vi "Ver 4.1.vi"() -> ()   [LabVIEW 2016]
doc: "This example VI shows how to use thermocouples to take a temperature measurement.\n\nNote:\nFor front panel measurements, make sure the Input switch is in the out position(F)\nFor plug-in card measurements, make sure the Input switch is in the in poisition(R)"
uses:
  Documents/keithley_27xx/Keithley 27XX/Public/Configure/Measurement Specific/Configure FRTD.vi
  Documents/keithley_27xx/Keithley 27XX/Public/Configure/Measurement Specific/Configure Thermocouple.vi
  Documents/keithley_27xx/Keithley 27XX/Public/Configure/Measurement Specific/Configure Thermistor.vi
  Documents/keithley_27xx/Keithley 27XX/Public/Data/Read Multiple Direct.vi
  <vilib>/Utility/file.llb/Write Delimited Spreadsheet (DBL).vi
  Documents/keithley_27xx/Keithley 27XX/Keithley 27XX.lvlib
panel:
  in  "Delay (s)":dbl
  in  "Notes":string
  in  "Number of Channels\nMeasured":dbl=3.0
  in  "Sensor Name 2":string
  in  "Sensor Name 1":string
  in  "Sensor Name 0":string
  out "XY Graph":cluster{dbl[], dbl[]}[](graph)
  out "Timestamp 2":dbl[](array[numeric])
  out "Timestamp 1":dbl[](array[numeric])
  out "Timestamp 0":dbl[](array[numeric])
  out "Case 2":dbl[](array[numeric])
  out "Case 1":dbl[](array[numeric])
  in  "Channel (2)":string="103"
  in  "Alpha2":dbl=0.0038
  in  "Beta2":dbl=0.1
  in  "Delta2 3":dbl=1.0
  in  "Sensor Type 2":string(combo)="Thermistor"
  in  "Channel (1)":string="102"
  in  "Alpha1":dbl=0.0038
  in  "Beta1":dbl=0.1
  in  "Delta1 2":dbl=1.0
  in  "Sensor Type 1":string(combo)="Thermistor"
  in  "Sensor Type 0":string(combo)="Thermistor"
  in  "Delta0":dbl=1.0
  in  "Beta0":dbl=0.1
  in  "Alpha0":dbl=0.0038
  in  "Serial Configuration":T1={"Baud Rate (9600)"=9600, "Flow Control (1: XON/XOFF)"=1, "Termination Char (0:CR)"=0} {"Termination Char (0:CR)" items=["CR", "LF", "CRLF (Do not use)", "LFCR (Do not use)"]; "Flow Control (1: XON/XOFF)" items=["None", "XON/XOFF", "RTS/CTS (2701 Only)", "XON/XOFF & RTS/CTS (2701 Only)"]; "Baud Rate (9600)" items=["300"=300, "600"=600, "1200"=1200, "2400"=2400, "4800"=4800, "9600"=9600, "19.2k"=19200, "38.4k (2701 Only)"=38400, "57.6k (2701 Only)"=57600, "115.2k (2701 Only)"=115200]}
  in  "VISA resource name":refnum<visa-resource-name>="TCPIP0::192.168.69.200::1394::SOCKET"
  in  "stop":bool
  out "Case 0":dbl[](array[numeric])
  in  "Channel (0)":string="101"
  in  "Temperature (0: Celsius)":u16(ring) items=["Celsius", "Fahrenheit", "Kelvin"]
  # "This is the delay in seconds \nbetween measuring. Note \nthat 0 is the fastest setting"
  # "Use this stop unless it is an emergency.\nUse the stop sign in the tool bar if \nthere is a danger from proceeding."
  # "*For front panel measurements, make sure the Input switch is in the out position(F)*\n  For plug-in card measurements, make sure the Input switch is in the in position(R)"
  # "© 2005 National Instruments Corporation.  ALL RIGHTS RESERVED."
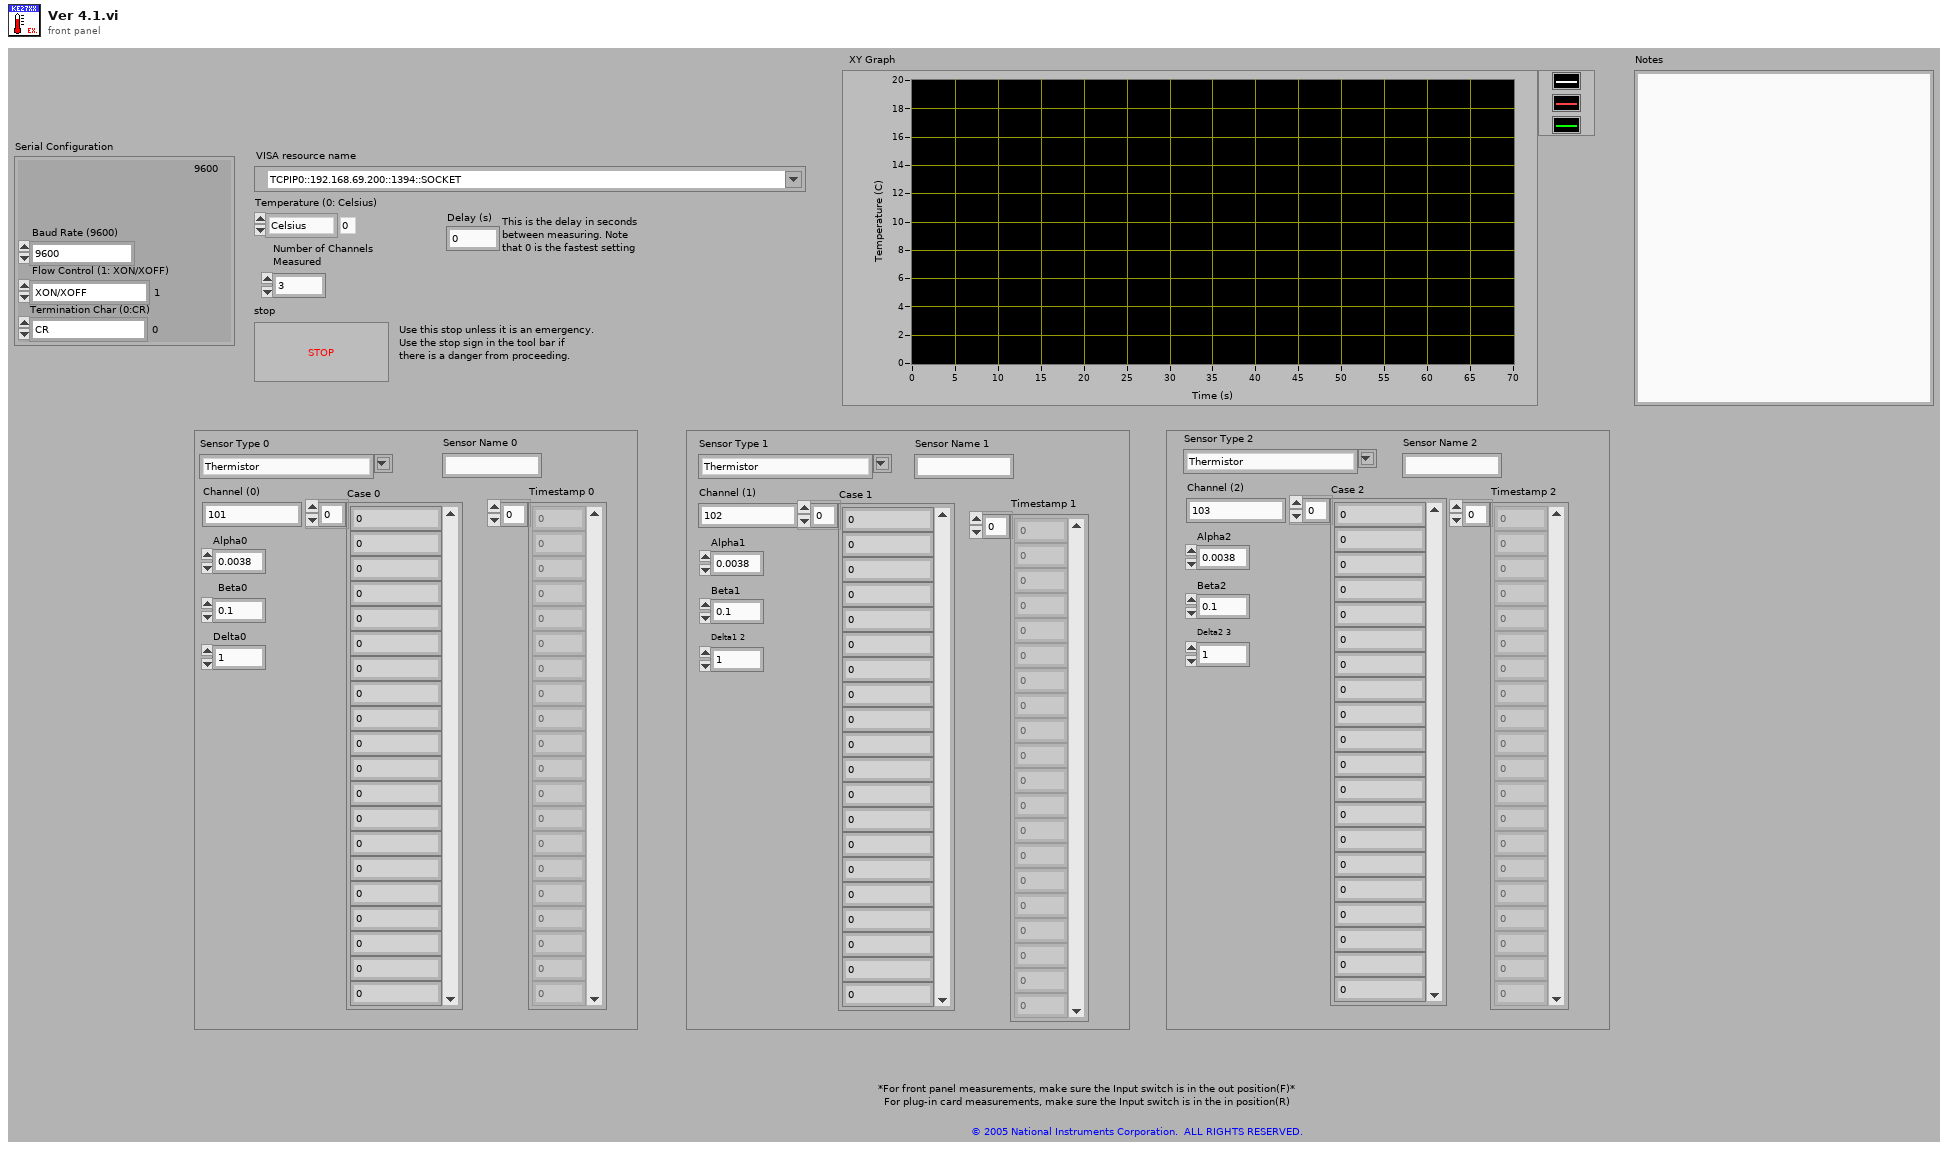
[diagram p1: front panel]
types:
  T1 = cluster{"Baud Rate (9600)":u32, "Flow Control (1: XON/XOFF)":u16, "Termination Char (0:CR)":u16}
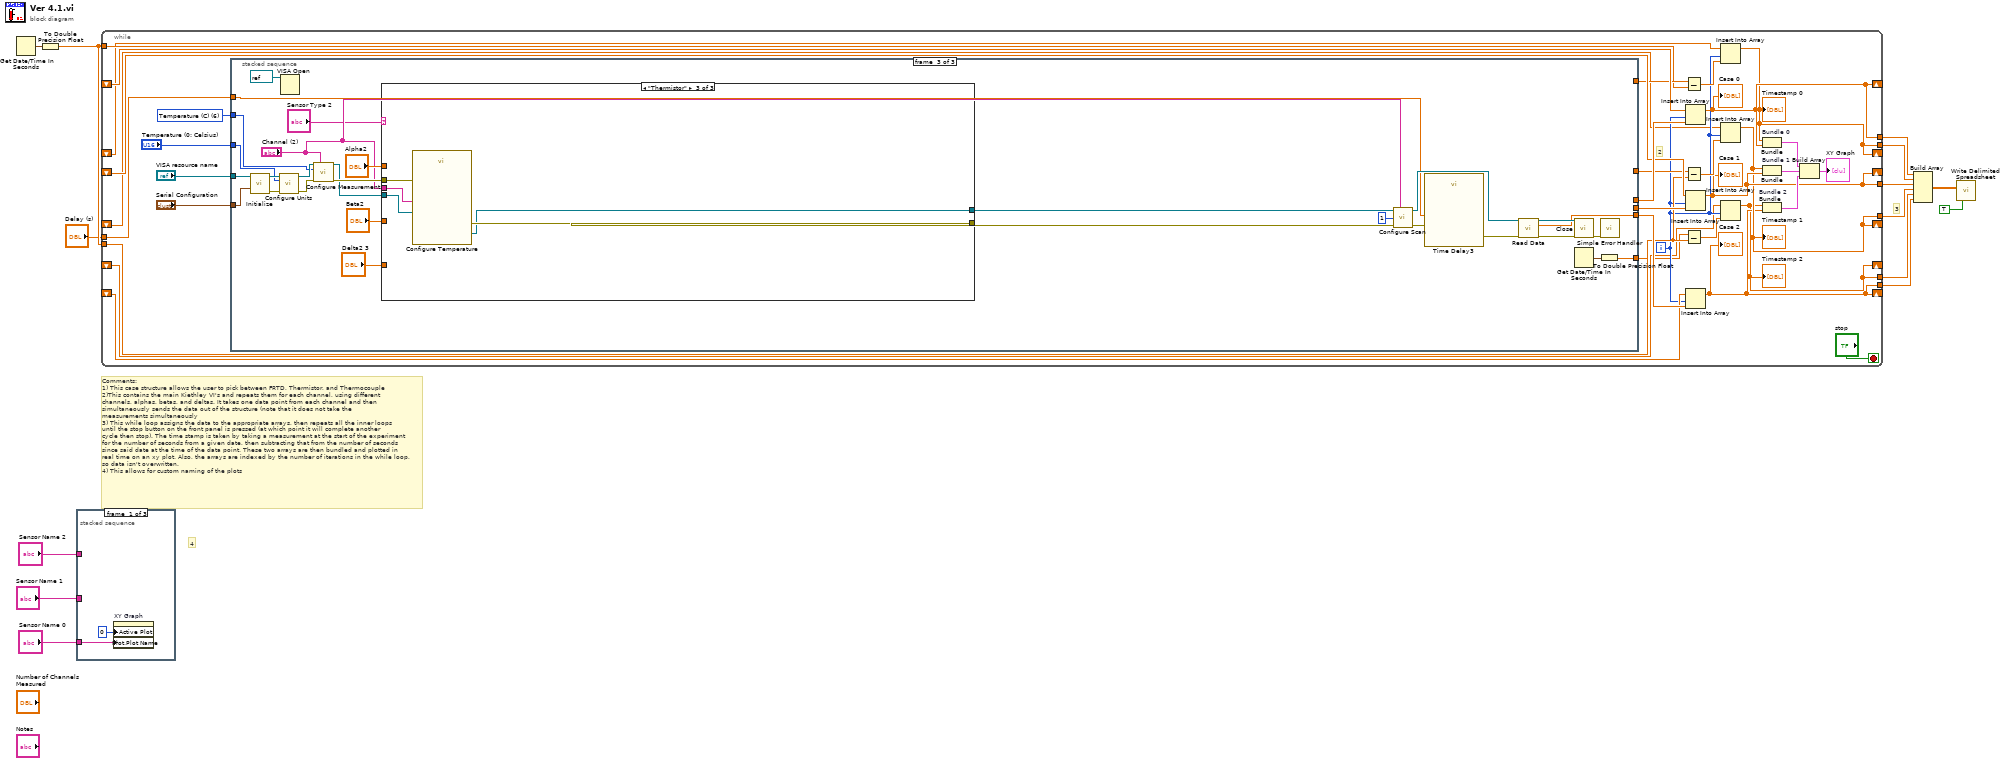
[diagram p0: block diagram]
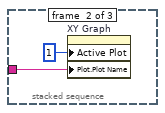
[diagram p2: hidden frame]
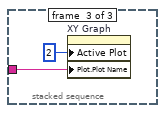
[diagram p3: hidden frame]
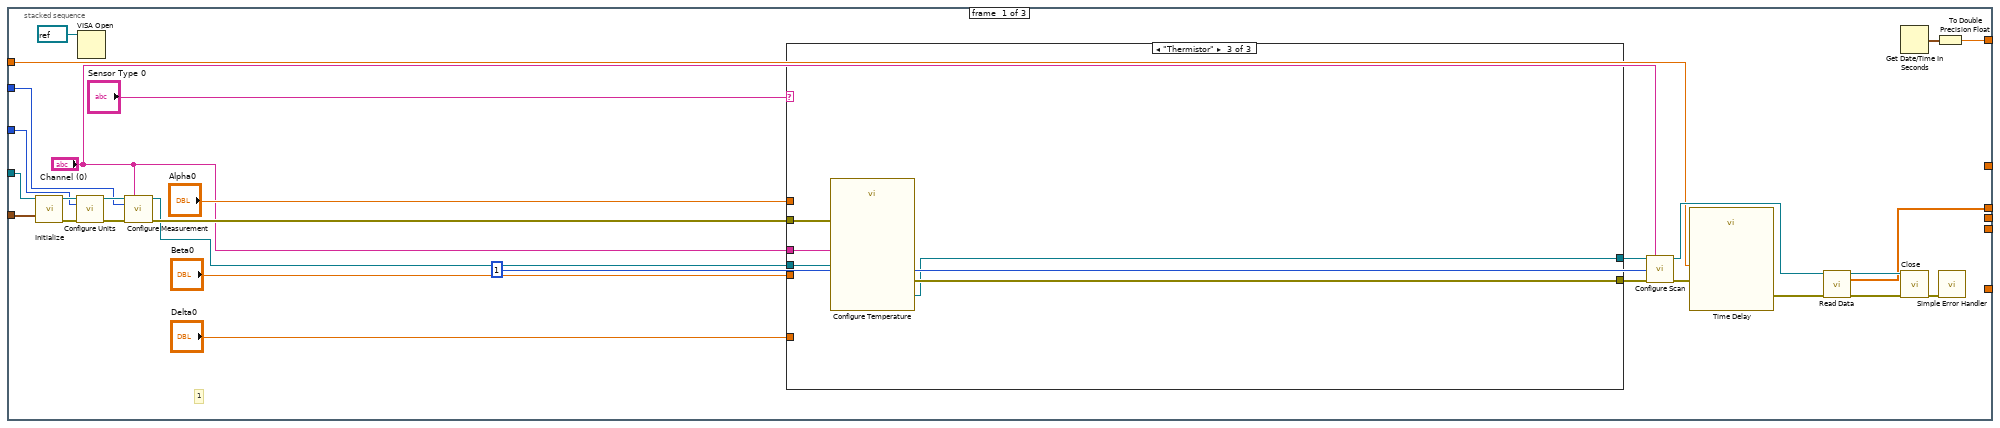
[diagram p4: hidden frame]
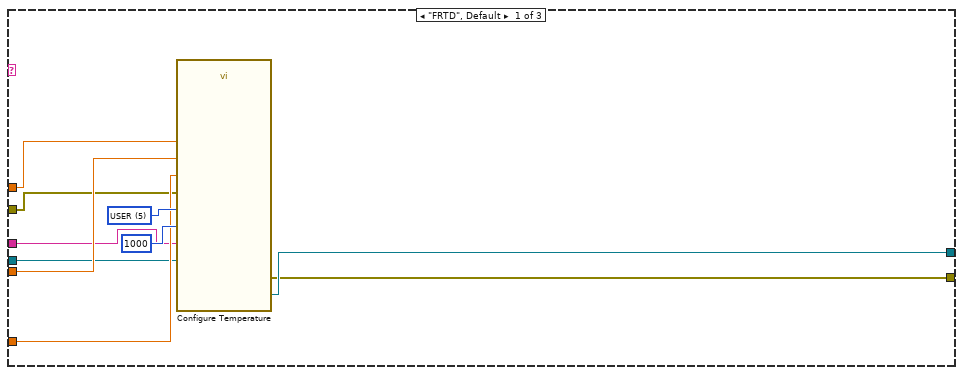
[diagram p5: hidden frame]
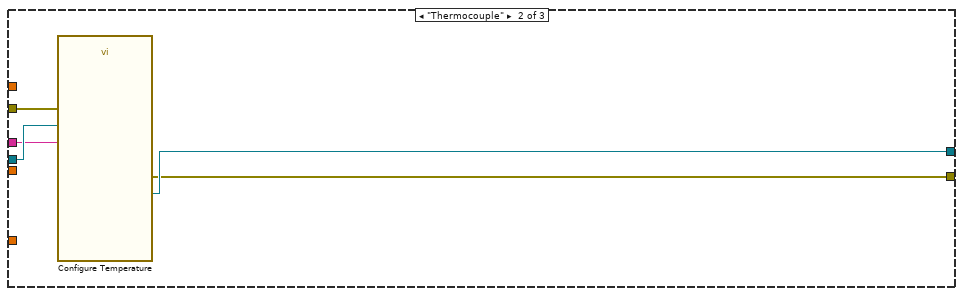
[diagram p6: hidden frame]
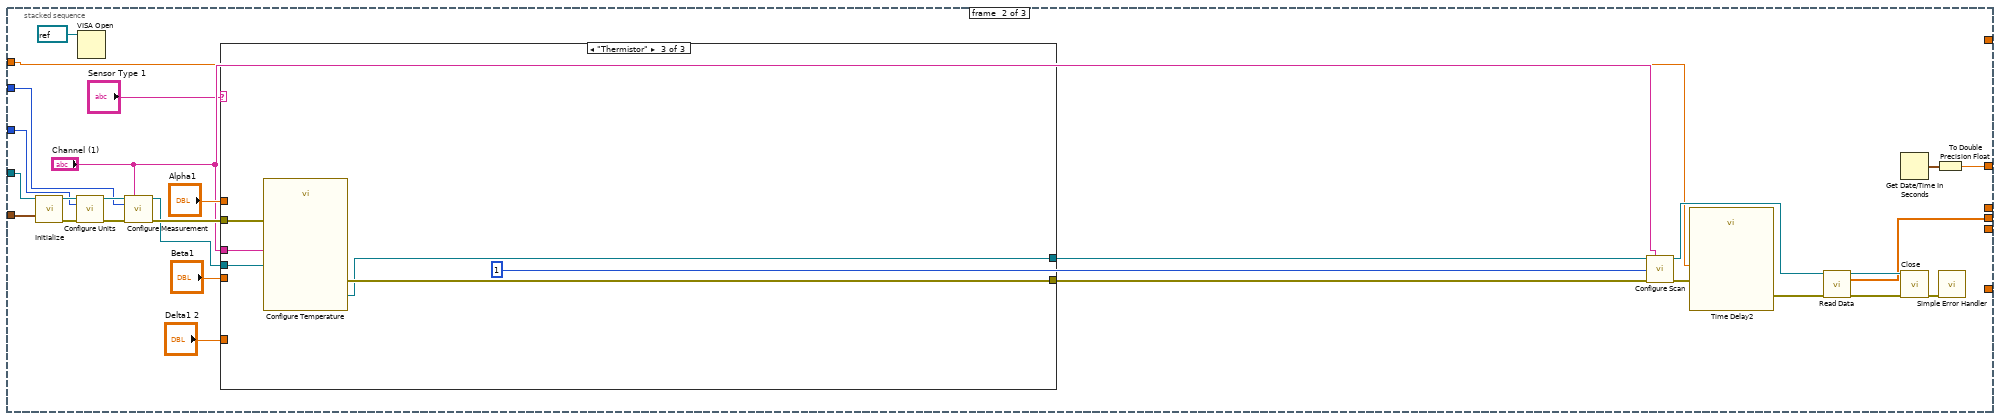
[diagram p7: hidden frame]
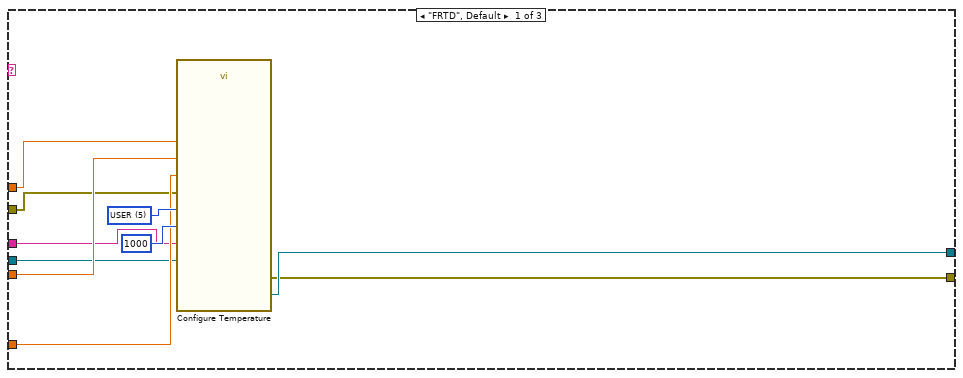
[diagram p8: hidden frame]
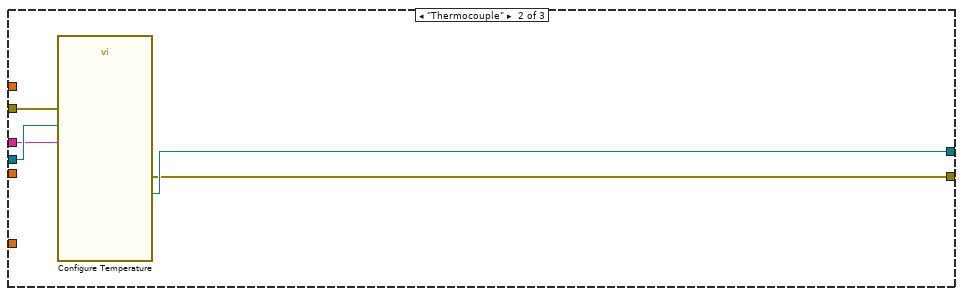
[diagram p9: hidden frame]
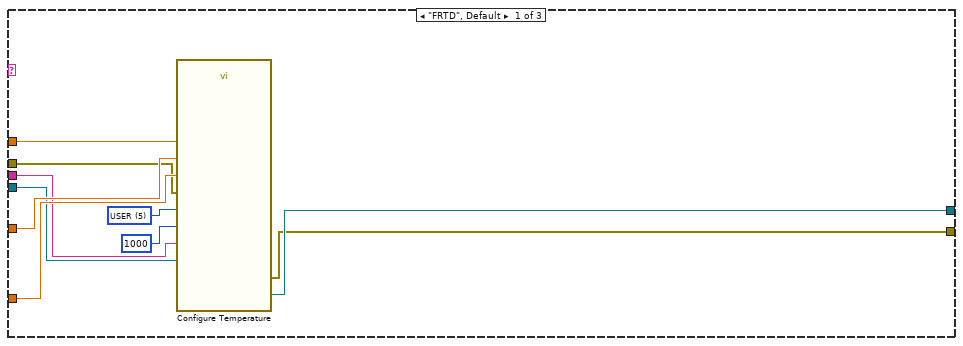
[diagram p10: hidden frame]
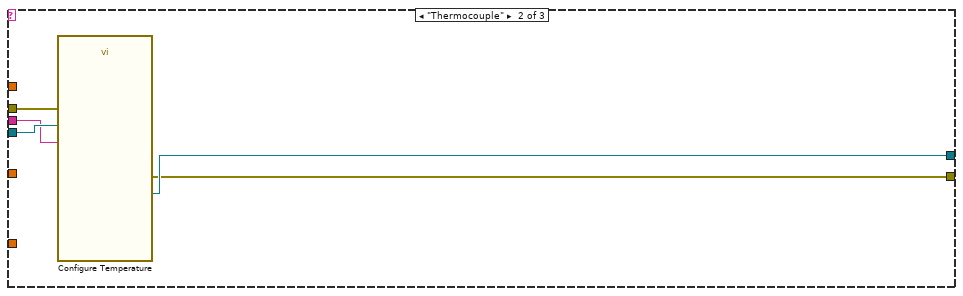
[diagram p11: hidden frame]
diagram:
  # "Comments:\n1) This case structure allows the user to pick between FRTD, Thermistor, and Thermocouple\n2)This contains the main Kiethley VI's and repeats them for each channel, using different\nchannels, alphas, betas, and deltas. It takes one data point from each channel and then \nsimultaneously sends the data out of the structure (note that it does not take the\nmeasurements simultaneously\n3) This while loop assigns the data to the appropriate arrays, then repeats all the inner loops\nuntil the stop button on the front panel is pressed (at which point it will complete another\ncycle then stop). The time stamp is taken by taking a measurement at the start of the experiment\nfor the number of seconds from a given date, then subtracting that from the number of seconds\nsince said date at the time of the data point. These two arrays are then bundled and plotted in\nreal time on an xy plot. Also, the arrays are indexed by the number of iterations in the while loop,\nso data isn't overwritten.\n4) This allows for custom naming of the plots"
  # "4"
  # "3"
  n1 = Get Date/Time In Seconds() -> (seconds since 1Jan1904=w14:timestamp)
  n2 = To Double Precision Float(number=w14) -> (double precision float=w13:dbl)
  n3 = stacked-sequence {
    tunnel: "Sensor Name 2" -> [_ _ w19]
    tunnel: "Sensor Name 0" -> [w15 _ _]
    tunnel: "Sensor Name 1" -> [_ w17 _]
    frame #0 {
      n4 = property on="XY Graph" class="XYGraph (strict)"("Active Plot"=0, "Plot.Plot Name"=w15) -> ()  [unwired: 2 in, 2 out]
    }
    frame #1 {
      n5 = property on="XY Graph" class="XYGraph (strict)"("Active Plot"=1, "Plot.Plot Name"=w17) -> ()  [unwired: 2 in, 2 out]
    }
    frame #2 {
      n6 = property on="XY Graph" class="XYGraph (strict)"("Active Plot"=2, "Plot.Plot Name"=w19) -> ()  [unwired: 2 in, 2 out]
    }
  }
  n7 = while {
    shift-right: [w26] -> _
    shift-left: _ -> [w48]
    shift-right: [w24] -> _
    shift-left: _ -> [w46]
    shift-right: [w22] -> _
    shift-left: _ -> [w44]
    tunnel: w13 -> [w42]
    shift-right: [w25] -> _
    shift-left: _ -> [w40]
    tunnel: w13 -> [w38]
    shift-right: [w23] -> _
    shift-left: _ -> [w34]
    shift-right: [w21] -> _
    shift-left: _ -> [w33]
    tunnel: "Delay (s)" -> [w29]
    tunnel: [w26] -> w8
    tunnel: [w25] -> w7
    tunnel: [w24] -> w6
    tunnel: [w23] -> w5
    tunnel: [w22] -> w3
    tunnel: [w21] -> w4
    i -> [w36]
    stop <- "stop" stop-if-true
    w52 = u16 6 items=["DC Voltage", "AC Voltage", "DC Current", "AC Current", "Resistance", "Four-Wire Resistance", "Temperature (C)", "Frequency", "Period", "Continuity"] ("Function (0: DC Voltage)")
    # "2"
    n8 = stacked-sequence {
      tunnel: "VISA resource name" -> [w74 w123 w172]
      tunnel: "Serial Configuration" -> [w73 w122 w171]
      tunnel: w52 -> [w72 w121 w170]
      tunnel: "Temperature (0: Celsius)" -> [w71 w120 w169]
      tunnel: [w60 _ _] -> w50
      tunnel: [_ w109 _] -> w47
      tunnel: [_ _ w158] -> w45
      tunnel: [w58 _ _] -> w43
      tunnel: [_ w107 _] -> w39
      tunnel: [_ _ w156] -> w32
      tunnel: w29 -> [w55 w104 w153]
      frame #0 {
        # "1"
        n9 = call "Initialize.vi"("VISA resource name"=w74, "Serial Configuration"=w73) -> ("VISA resource name out"=w82:refnum<visa-resource-name>, "error out"=w77:errorcluster)  [unwired: 12 in]
        n10 = call "Configure Units.vi"("VISA resource name"=w82, "Temperature (0: Celsius)"=w71, "error in (no error)"=w77) -> ("VISA resource name out"=w83:refnum<visa-resource-name>, "error out"=w76:errorcluster)  [unwired: 11 in]
        n11 = VISA Open(VISA resource name=refnum<visa-resource-name> refnum) -> ()  [unwired: 4 in, 2 out]
        n12 = call "Configure Measurement.vi"("VISA resource name"=w83, "Scan List (Empty)"="Channel (0)", "Function (0: DC Voltage)"=w72, "error in (no error)"=w76) -> ("VISA resource name out"=w64:refnum<visa-resource-name>, "error out"=w65:errorcluster)  [unwired: 10 in]
        n13 = case shown="\"Thermistor\"" "Sensor Type 0" {
          tunnel: [w92 w97 w103] -> w70
          tunnel: [w93 w98 w102] -> w69
          tunnel: "Delta0" -> [w87 _ _]
          tunnel: "Beta0" -> [w88 _ _]
          tunnel: "Alpha0" -> [w89 _ _]
          tunnel: w65 -> [w86 w96 w99]
          tunnel: w64 -> [w85 w95 w100]
          tunnel: "Channel (0)" -> [w84 w94 w101]
          frame "FRTD", Default {
            w91 = u16 5 items=["PT100", "D100", "F100", "PT3916", "PT385", "USER"] ("FRTD Type (0: PT100)")
            n14 = call-poly "Configure Temperature.vi"("VISA resource name"=w85, "FRTD Type (0: PT100)"=w91, "error in (no error)"=w86, "Scan List (Empty)"=w84, "R Zero (100)"=1000, "Alpha (0.00385)"=w89, "Beta (0.111)"=w88, "Delta (1.507)"=w87) -> ("VISA resource name out"=w93:refnum<visa-resource-name>, "error out"=w92:errorcluster)  [unwired: 10 in]
          }
          frame "Thermocouple" {
            n15 = call-poly "Configure Temperature.vi"("VISA resource name"=w95, "error in (no error)"=w96, "Scan List (Empty)"=w94) -> ("VISA resource name out"=w98:refnum<visa-resource-name>, "error out"=w97:errorcluster)  [unwired: 15 in]
          }
          frame "Thermistor" {
            n16 = call-poly "Configure Temperature.vi"("VISA resource name"=w100, "error in (no error)"=w99, "Scan List (Empty)"=w101) -> ("VISA resource name out"=w102:refnum<visa-resource-name>, "error out"=w103:errorcluster)  [unwired: 15 in]
          }
        }
        n17 = call "Configure Scan.vi"("VISA resource name"=w69, "Channel List (101:110)"="Channel (0)", "Sample Count (100)"=1, "error in (no error)"=w70) -> ("VISA resource name out"=w80:refnum<visa-resource-name>, "error out"=w57:errorcluster)  [unwired: 10 in]
        n18 = call "Time Delay"("error in (no error)"=w57, "Delay Time (s)"=w55) -> ("error out"=w56:errorcluster)  [unwired: 9 in]
        n19 = call-poly "Read Data.vi"("VISA resource name"=w80, "error in (no error)"=w56) -> ("VISA resource name out"=w78:refnum<visa-resource-name>, "Measurement Data"=w60:dbl[], "error out"=w79:errorcluster)  [unwired: 8 in, 3 out]
        n20 = Get Date/Time In Seconds() -> (seconds since 1Jan1904=w59:timestamp)
        n21 = call "Close.vi"("VISA resource name"=w78, "error in (no error)"=w79) -> ("error out"=w81:errorcluster)  [unwired: 13 in]
        n22 = To Double Precision Float(number=w59) -> (double precision float=w58:dbl)
        n23 = call <vilib>:"Simple Error Handler.vi"("error in (no error)"=w81) -> ()  [unwired: 4 in, 5 out]
      }
      frame #1 {
        n24 = call "Initialize.vi"("VISA resource name"=w123, "Serial Configuration"=w122) -> ("VISA resource name out"=w131:refnum<visa-resource-name>, "error out"=w126:errorcluster)  [unwired: 12 in]
        n25 = call "Configure Units.vi"("VISA resource name"=w131, "Temperature (0: Celsius)"=w120, "error in (no error)"=w126) -> ("VISA resource name out"=w132:refnum<visa-resource-name>, "error out"=w125:errorcluster)  [unwired: 11 in]
        n26 = VISA Open(VISA resource name=refnum<visa-resource-name> refnum) -> ()  [unwired: 4 in, 2 out]
        n27 = call "Configure Measurement.vi"("VISA resource name"=w132, "Scan List (Empty)"="Channel (1)", "Function (0: DC Voltage)"=w121, "error in (no error)"=w125) -> ("VISA resource name out"=w113:refnum<visa-resource-name>, "error out"=w114:errorcluster)  [unwired: 10 in]
        n28 = case shown="\"Thermistor\"" "Sensor Type 1" {
          tunnel: [w141 w146 w152] -> w119
          tunnel: [w142 w147 w151] -> w118
          tunnel: "Delta1 2" -> [w136 _ _]
          tunnel: "Beta1" -> [w137 _ _]
          tunnel: "Alpha1" -> [w138 _ _]
          tunnel: w114 -> [w135 w145 w148]
          tunnel: w113 -> [w134 w144 w149]
          tunnel: "Channel (1)" -> [w133 w143 w150]
          frame "FRTD", Default {
            w140 = u16 5 items=["PT100", "D100", "F100", "PT3916", "PT385", "USER"] ("FRTD Type (0: PT100)")
            n29 = call-poly "Configure Temperature.vi"("VISA resource name"=w134, "FRTD Type (0: PT100)"=w140, "error in (no error)"=w135, "Scan List (Empty)"=w133, "R Zero (100)"=1000, "Alpha (0.00385)"=w138, "Beta (0.111)"=w137, "Delta (1.507)"=w136) -> ("VISA resource name out"=w142:refnum<visa-resource-name>, "error out"=w141:errorcluster)  [unwired: 10 in]
          }
          frame "Thermocouple" {
            n30 = call-poly "Configure Temperature.vi"("VISA resource name"=w144, "error in (no error)"=w145, "Scan List (Empty)"=w143) -> ("VISA resource name out"=w147:refnum<visa-resource-name>, "error out"=w146:errorcluster)  [unwired: 15 in]
          }
          frame "Thermistor" {
            n31 = call-poly "Configure Temperature.vi"("VISA resource name"=w149, "error in (no error)"=w148, "Scan List (Empty)"=w150) -> ("VISA resource name out"=w151:refnum<visa-resource-name>, "error out"=w152:errorcluster)  [unwired: 15 in]
          }
        }
        n32 = call "Configure Scan.vi"("VISA resource name"=w118, "Channel List (101:110)"="Channel (1)", "Sample Count (100)"=1, "error in (no error)"=w119) -> ("VISA resource name out"=w129:refnum<visa-resource-name>, "error out"=w106:errorcluster)  [unwired: 10 in]
        n33 = call "Time Delay2"("error in (no error)"=w106, "Delay Time (s)"=w104) -> ("error out"=w105:errorcluster)  [unwired: 9 in]
        n34 = call-poly "Read Data.vi"("VISA resource name"=w129, "error in (no error)"=w105) -> ("VISA resource name out"=w127:refnum<visa-resource-name>, "Measurement Data"=w109:dbl[], "error out"=w128:errorcluster)  [unwired: 8 in, 3 out]
        n35 = Get Date/Time In Seconds() -> (seconds since 1Jan1904=w108:timestamp)
        n36 = call "Close.vi"("VISA resource name"=w127, "error in (no error)"=w128) -> ("error out"=w130:errorcluster)  [unwired: 13 in]
        n37 = To Double Precision Float(number=w108) -> (double precision float=w107:dbl)
        n38 = call <vilib>:"Simple Error Handler.vi"("error in (no error)"=w130) -> ()  [unwired: 4 in, 5 out]
      }
      frame #2 {
        n39 = call "Initialize.vi"("VISA resource name"=w172, "Serial Configuration"=w171) -> ("VISA resource name out"=w180:refnum<visa-resource-name>, "error out"=w175:errorcluster)  [unwired: 12 in]
        n40 = call "Configure Units.vi"("VISA resource name"=w180, "Temperature (0: Celsius)"=w169, "error in (no error)"=w175) -> ("VISA resource name out"=w181:refnum<visa-resource-name>, "error out"=w174:errorcluster)  [unwired: 11 in]
        n41 = VISA Open(VISA resource name=refnum<visa-resource-name> refnum) -> ()  [unwired: 4 in, 2 out]
        n42 = call "Configure Measurement.vi"("VISA resource name"=w181, "Scan List (Empty)"="Channel (2)", "Function (0: DC Voltage)"=w170, "error in (no error)"=w174) -> ("VISA resource name out"=w162:refnum<visa-resource-name>, "error out"=w163:errorcluster)  [unwired: 10 in]
        n43 = case shown="\"Thermistor\"" "Sensor Type 2" {
          tunnel: [w190 w195 w201] -> w168
          tunnel: [w191 w196 w200] -> w167
          tunnel: "Delta2 3" -> [w185 _ _]
          tunnel: "Beta2" -> [w186 _ _]
          tunnel: "Alpha2" -> [w187 _ _]
          tunnel: w163 -> [w184 w194 w197]
          tunnel: w162 -> [w183 w193 w198]
          tunnel: "Channel (2)" -> [w182 w192 w199]
          frame "FRTD", Default {
            w189 = u16 5 items=["PT100", "D100", "F100", "PT3916", "PT385", "USER"] ("FRTD Type (0: PT100)")
            n44 = call-poly "Configure Temperature.vi"("VISA resource name"=w183, "FRTD Type (0: PT100)"=w189, "error in (no error)"=w184, "Scan List (Empty)"=w182, "R Zero (100)"=1000, "Alpha (0.00385)"=w187, "Beta (0.111)"=w186, "Delta (1.507)"=w185) -> ("VISA resource name out"=w191:refnum<visa-resource-name>, "error out"=w190:errorcluster)  [unwired: 10 in]
          }
          frame "Thermocouple" {
            n45 = call-poly "Configure Temperature.vi"("VISA resource name"=w193, "error in (no error)"=w194, "Scan List (Empty)"=w192) -> ("VISA resource name out"=w196:refnum<visa-resource-name>, "error out"=w195:errorcluster)  [unwired: 15 in]
          }
          frame "Thermistor" {
            n46 = call-poly "Configure Temperature.vi"("VISA resource name"=w198, "error in (no error)"=w197, "Scan List (Empty)"=w199) -> ("VISA resource name out"=w200:refnum<visa-resource-name>, "error out"=w201:errorcluster)  [unwired: 15 in]
          }
        }
        n47 = call "Configure Scan.vi"("VISA resource name"=w167, "Channel List (101:110)"="Channel (2)", "Sample Count (100)"=1, "error in (no error)"=w168) -> ("VISA resource name out"=w178:refnum<visa-resource-name>, "error out"=w155:errorcluster)  [unwired: 10 in]
        n48 = call "Time Delay3"("error in (no error)"=w155, "Delay Time (s)"=w153) -> ("error out"=w154:errorcluster)  [unwired: 9 in]
        n49 = call-poly "Read Data.vi"("VISA resource name"=w178, "error in (no error)"=w154) -> ("VISA resource name out"=w176:refnum<visa-resource-name>, "Measurement Data"=w158:dbl[], "error out"=w177:errorcluster)  [unwired: 8 in, 3 out]
        n50 = call "Close.vi"("VISA resource name"=w176, "error in (no error)"=w177) -> ("error out"=w179:errorcluster)  [unwired: 13 in]
        n51 = Get Date/Time In Seconds() -> (seconds since 1Jan1904=w157:timestamp)
        n52 = To Double Precision Float(number=w157) -> (double precision float=w156:dbl)
        n53 = call <vilib>:"Simple Error Handler.vi"("error in (no error)"=w179) -> ()  [unwired: 4 in, 5 out]
      }
    }
    n54 = Subtract(x=w43, y=w42) -> (x-y=w41:dbl)
    n55 = Subtract(x=w39, y=w38) -> (x-y=w37:dbl)
    n56 = Subtract(x=w32, y=w38) -> (x-y=w35:dbl)
    n57 = Insert Into Array(array=w48, index=w36, new element=w50) -> (w26:dbl[])
    "Case 0" <- w26
    n58 = Insert Into Array(array=w46, index=w36, new element=w47) -> (w24:dbl[])
    "Case 1" <- w24
    n59 = Insert Into Array(array=w44, index=w36, new element=w45) -> (w22:dbl[])
    "Case 2" <- w22
    n60 = Insert Into Array(array=w40, index=w36, new element=w41) -> (w25:dbl[])
    "Timestamp 0" <- w25
    n61 = Insert Into Array(array=w34, index=w36, new element=w37) -> (w23:dbl[])
    "Timestamp 1" <- w23
    n62 = Insert Into Array(array=w33, index=w36, new element=w35) -> (w21:dbl[])
    "Timestamp 2" <- w21
    n63 = Bundle "Bundle 0"(w25, w26) -> (w27:cluster{dbl[], dbl[]})  [unwired: 1 in]
    n64 = Bundle "Bundle 1"(w23, w24) -> (w31:cluster{dbl[], dbl[]})  [unwired: 1 in]
    n65 = Bundle "Bundle 2"(w21, w22) -> (w30:cluster{dbl[], dbl[]})  [unwired: 1 in]
    n66 = Build Array(w27, w31, w30) -> (→"XY Graph":cluster{dbl[], dbl[]}[])
  }
  n67 = Build Array(w8, w7, w6, w5, w4, w3) -> (w2:dbl[][])
  n68 = call-poly <vilib>:"Write Delimited Spreadsheet.vi"("2D data"=w2, "transpose? (no:F)"=TRUE) -> ()  [unwired: 12 in, 2 out]
